vi "SDSU_Reg_Fields2Values.vi"(10 "Register":T1) -> (1 "binary string":string, 2 "Register out":T1)   [LabVIEW 2016]
uses:
  SDSU_Register.ctl
  SDSU_RegField.ctl
panel:
  out "error out":errorcluster
  in  "error in (no error)":errorcluster
  out "hex integer string":string
  out "value":i32
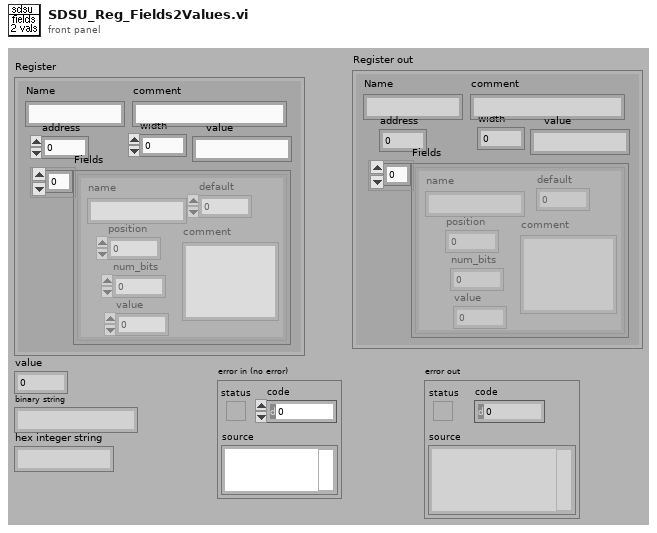
[diagram p1: front panel]
types:
  T1 = typedef "SDSU_Register.ctl" = cluster{"Name":string, "address":i16, "width":i16, "comment":string, "Fields":T2[], "value":string}
  T2 = typedef "SDSU_RegField.ctl" = cluster{"name":string, "position":u16, "num_bits":u16, "default":i16, "comment":string, "value":i32}
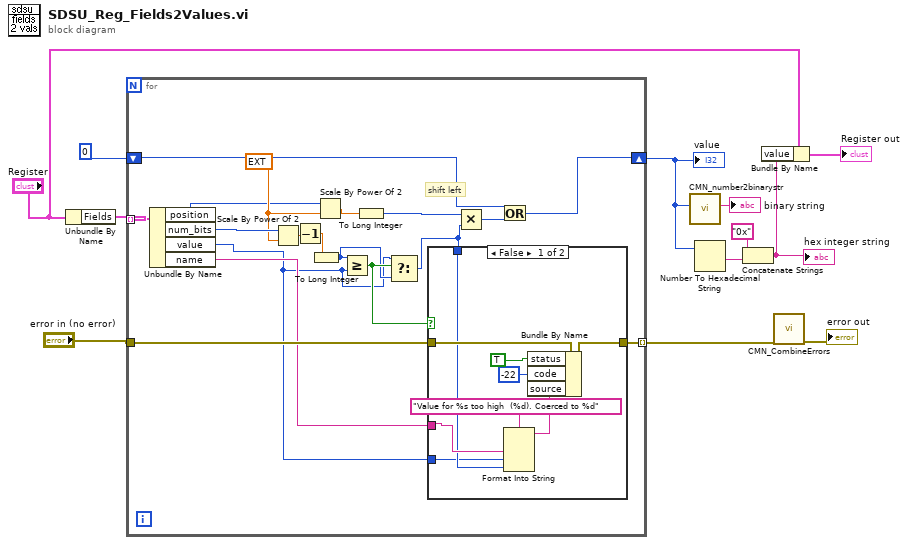
[diagram p0: block diagram]
diagram:
  n1 = Unbundle By Name("Register") -> ("Fields"=w12:T2[])
  n2 = for {
    tunnel: w12 -> [w30] mode=indexing
    shift-right: [w21] -> w10
    shift-left: 0 -> [w22]
    tunnel: "error in (no error)" -> [w20]
    tunnel: [w19] -> w2 mode=indexing
    w27 = ext 1.0 ("x")
    # "shift left"
    n3 = Unbundle By Name(w30) -> ("position"=w26:u16, "num_bits"=w29:u16, "value"=w13:i32, "name"=w18:string)
    n4 = Scale By Power Of 2(n=w29, x=w27) -> (x*2^n=w28:ext)
    n5 = Decrement(x=w28) -> (x-1=w17:ext)
    n6 = To Long Integer(number=w17) -> (32bit integer=w14:i32)
    n7 = Scale By Power Of 2(n=w26, x=w27) -> (x*2^n=w25:ext)
    n8 = Greater Or Equal?(x=w14, y=w13) -> (x >= y?=w16:bool)
    n9 = To Long Integer(number=w25) -> (32bit integer=w23:i32)
    n10 = Select(t=w13, s=w16, f=w14) -> (s? t:f=w15:i32)
    n11 = case shown="False" w16 {
      tunnel: w20 -> [w39 w40]
      tunnel: [w38 w40] -> w19
      tunnel: w18 -> [w34 _]
      tunnel: w13 -> [w31 _]
      tunnel: w15 -> [w32 _]
      frame False {
        n12 = Format Into String(format string="Value for %s too high  (%d). Coerced to %d", w34, w31, w32) -> (resulting string=w33:string)  [unwired: 2 in, 1 out]
        n13 = Bundle By Name(cluster=w39, "status"=TRUE, "code"=-22, "source"=w33) -> (w38:errorcluster)
      }
      frame True {
      }
    }
    n14 = Multiply(x=w23, y=w15) -> (x*y=w24:i32)
    n15 = Or(x=w22, y=w24) -> (x .or. y?=w21:i32)
  }
  "value" <- w10
  n16 = call "CMN_number2binarystr.vi"("decimal number"=w10) -> ("binary string"=→"binary string":string)  [unwired: 10 out]
  n17 = Number To Hexadecimal String(2:w10) -> (0:w8:string)  [unwired: 1 out]
  n18 = Concatenate Strings("0x" ("string"), w8) -> (w3:string)
  "hex integer string" <- w3
  n19 = Bundle By Name(cluster="Register", "value"=w3) -> (→"Register out":T1)
  n20 = call "CMN_CombineErrors.vi"("Errors"=w2) -> ("error out"=→"error out":errorcluster)  [unwired: 10 out]
